vi "load_templates_subVI.vi"(8 "error in (no error)":errorcluster) -> (0 "error out":errorcluster, 1 "Lips Template":T1(plugin-control), 2 "Nose Template":T1(plugin-control), 3 "Eye Template":T1(plugin-control))   [LabVIEW 2013]
uses:
  <vilib>/vision/NI_Vision_Development_Module.lvlib
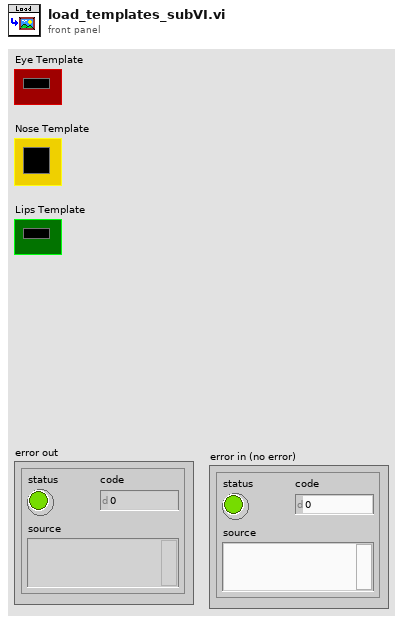
[diagram p1: front panel]
types:
  T1 = typedef "IMAQ Image.ctl" = refnum<image>
  T2 = typedef "Image Type" = u32
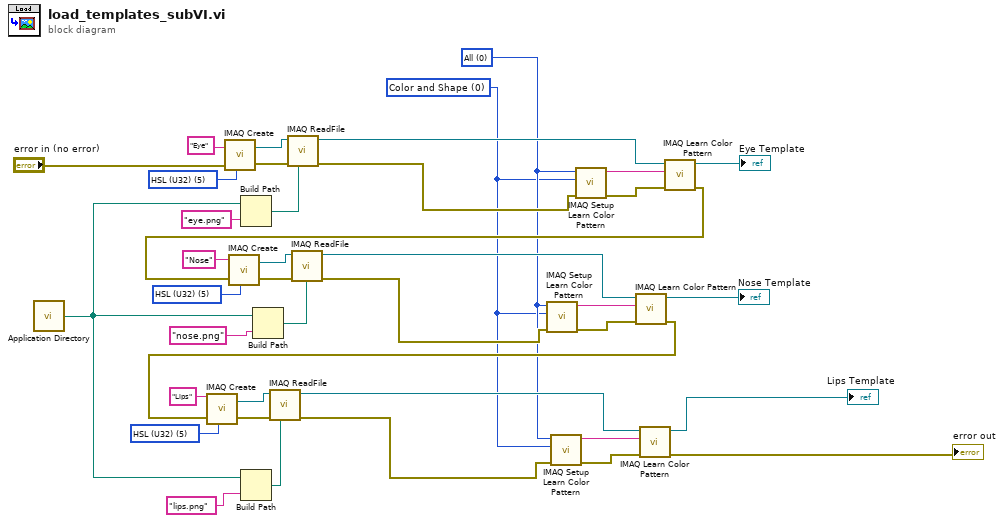
[diagram p0: block diagram]
diagram:
  w1 = u32 0 items=["Color and Shape", "Color", "Shape "] ("Feature Mode")
  w2 = u32 0 items=["All", "Shift Information", "Rotation Information"] ("Learn Mode")
  w11 = T2 5 items=["Grayscale (U8)", "Grayscale (I16)", "Grayscale (SGL)", "Complex (CSG)", "RGB (U32)", "HSL (U32)", "RGB (U64)", "Grayscale (U16)"] ("Image Type")
  w8 = T2 5 items=["Grayscale (U8)", "Grayscale (I16)", "Grayscale (SGL)", "Complex (CSG)", "RGB (U32)", "HSL (U32)", "RGB (U64)", "Grayscale (U16)"] ("Image Type")
  w4 = T2 5 items=["Grayscale (U8)", "Grayscale (I16)", "Grayscale (SGL)", "Complex (CSG)", "RGB (U32)", "HSL (U32)", "RGB (U64)", "Grayscale (U16)"] ("Image Type")
  n1 = call <vilib>:"Application Directory.vi"() -> ("Application Directory"=w37:path)
  n2 = call "IMAQ Create"("Image Name"="Eye", "Image Type"=w4, "error in (no error)"="error in (no error)") -> ("New Image"=w6:T1, "error out"=w5:errorcluster)  [unwired: 2 in]
  n3 = Build Path(base path=w37, name or relative path="eye.png") -> (appended path=w36:path)
  n4 = Build Path(base path=w37, name or relative path="lips.png") -> (appended path=w35:path)
  n5 = Build Path(base path=w37, name or relative path="nose.png") -> (appended path=w34:path)
  n6 = call "IMAQ ReadFile"("File Path"=w36, "error in (no error)"=w5, "Image"=w6) -> ("error out"=w26:errorcluster, "Image Out"=w15:T1)  [unwired: 4 in, 3 out]
  n7 = call "IMAQ Setup Learn Color Pattern"("error in (no error)"=w26, "Feature Mode"=w1, "Learn Mode"=w2) -> ("error out"=w13:errorcluster, "Learn Color Pattern Setup Data"=w14:string)  [unwired: 7 in]
  n8 = call "IMAQ Learn Color Pattern"("error in (no error)"=w13, "Learn Color Pattern Setup Data"=w14, "Image"=w15) -> ("error out"=w28:errorcluster, "Template Image Out"=→"Eye Template":T1)  [unwired: 7 in]
  n9 = call "IMAQ Create"("Image Name"="Nose", "Image Type"=w8, "error in (no error)"=w28) -> ("New Image"=w18:T1, "error out"=w7:errorcluster)  [unwired: 2 in]
  n10 = call "IMAQ ReadFile"("File Path"=w34, "error in (no error)"=w7, "Image"=w18) -> ("error out"=w25:errorcluster, "Image Out"=w22:T1)  [unwired: 4 in, 3 out]
  n11 = call "IMAQ Setup Learn Color Pattern"("error in (no error)"=w25, "Feature Mode"=w1, "Learn Mode"=w2) -> ("error out"=w17:errorcluster, "Learn Color Pattern Setup Data"=w16:string)  [unwired: 7 in]
  n12 = call "IMAQ Learn Color Pattern"("error in (no error)"=w17, "Learn Color Pattern Setup Data"=w16, "Image"=w22) -> ("error out"=w29:errorcluster, "Template Image Out"=→"Nose Template":T1)  [unwired: 7 in]
  n13 = call "IMAQ Create"("Image Name"="Lips", "Image Type"=w11, "error in (no error)"=w29) -> ("New Image"=w19:T1, "error out"=w12:errorcluster)  [unwired: 2 in]
  n14 = call "IMAQ ReadFile"("File Path"=w35, "error in (no error)"=w12, "Image"=w19) -> ("error out"=w24:errorcluster, "Image Out"=w23:T1)  [unwired: 4 in, 3 out]
  n15 = call "IMAQ Setup Learn Color Pattern"("error in (no error)"=w24, "Feature Mode"=w1, "Learn Mode"=w2) -> ("error out"=w20:errorcluster, "Learn Color Pattern Setup Data"=w21:string)  [unwired: 7 in]
  n16 = call "IMAQ Learn Color Pattern"("error in (no error)"=w20, "Learn Color Pattern Setup Data"=w21, "Image"=w23) -> ("error out"=→"error out":errorcluster, "Template Image Out"=→"Lips Template":T1)  [unwired: 7 in]
